vi "Wrapped To Absolute.vi"(8 "Desired Angle":dbl, 11 "Wrapped Value":dbl) -> (0 "x-y*floor(x/y)":dbl, 3 "Output":dbl)   [LabVIEW 2015]
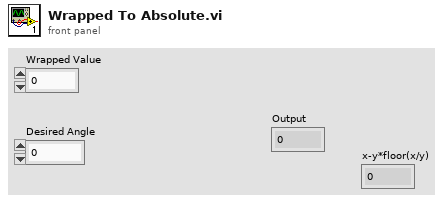
[diagram p1: front panel]
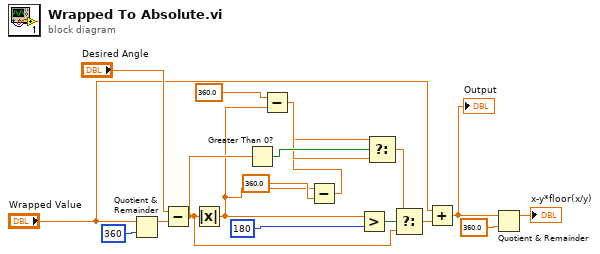
[diagram p0: block diagram]
diagram:
  n1 = Quotient & Remainder(x="Wrapped Value", y=360) -> (x-y*floor(x/y)=w16:dbl)  [unwired: 1 out]
  n2 = Subtract(x="Desired Angle", y=w16) -> (x-y=w5:dbl)
  n3 = Absolute Value(x=w5) -> (abs(x)=w3:dbl)
  n4 = Greater Than 0?(x=w5) -> (x > 0?=w7:bool)
  n5 = Subtract(x=360.0, y=w3) -> (x-y=w6:dbl)
  n6 = Subtract(x=w3, y=360.0 ("x")) -> (x-y=w2:dbl)
  n7 = Greater?(x=w3, y=180) -> (0:w15:bool)
  n8 = Select(t=w2, s=w7, f=w6) -> (s? t:f=w1:dbl)
  n9 = Select(t=w1, s=w15, f=w5) -> (s? t:f=w12:dbl)
  n10 = Add(x="Wrapped Value", y=w12) -> (x+y=w10:dbl)
  "Output" <- w10
  n11 = Quotient & Remainder(x=w10, y=360.0) -> (x-y*floor(x/y)=→"x-y*floor(x/y)":dbl)  [unwired: 1 out]
